vi "Read Attributes Metadata.vi"(11 "Base Attributes in":refnum<class "Base Attributes.lvclass">) -> (2 "Attributes Metadata":refnum<class "Attributes Metadata.lvclass">)   [LabVIEW 2020, in "jettl.lvlib" / "Base Attributes.lvlib" / "Base Attributes.lvclass"]
uses:
  Base Attributes.lvclass
  Base Attributes.lvclass/Base Attributes.ctl
  Attributes Metadata/Attributes Metadata.lvclass
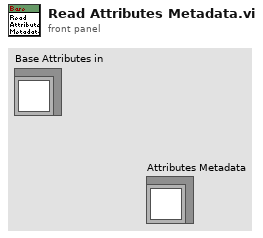
[diagram p1: front panel]
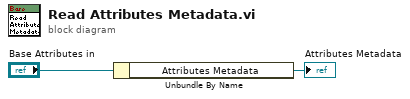
[diagram p0: block diagram]
diagram:
  n1 = Unbundle By Name("Base Attributes in") -> ("Attributes Metadata"=→"Attributes Metadata":refnum<class "Attributes Metadata.lvclass">)
